vi "test_Multiple Global Type Cast Single Channel Command Message using Trigger and Padding.vi"(8 "error in (no error)":errorcluster, 11 "TestCase in":refnum<class "Instrument Addon Common System Tests.lvclass">) -> (0 "error out":errorcluster, 3 "TestCase out":refnum<class "Instrument Addon Common System Tests.lvclass">)   [LabVIEW 2019, in "Instrument Addon Common System Tests.lvclass"]
uses:
  Instrument Addon Common System Tests.lvclass
  C:/Program Files (x86)/National Instruments/LabVIEW 2019/vi.lib/NI/VeriStand Custom Device Testing Tools/VeriStandTestCase/VeriStandTestCase.lvclass
  <vilib>/NI VeriStand/Execution/Workspace/NI VeriStand - Set Multiple Channel Values.vi
  <vilib>/NI VeriStand/Execution/Workspace/NI VeriStand - Get Multiple Channel Values.vi
  <vilib>/addons/_JKI Toolkits/VI Tester/TestCase.llb/TestCase.lvclass
  <vilib>/NI VeriStand/Execution/Workspace/NI_VS Workspace ExecutionAPI.lvlib
  C:/Program Files (x86)/National Instruments/LabVIEW 2019/vi.lib/addons/_JKI Toolkits/VI Tester/TestCase.llb/TestCase.lvclass
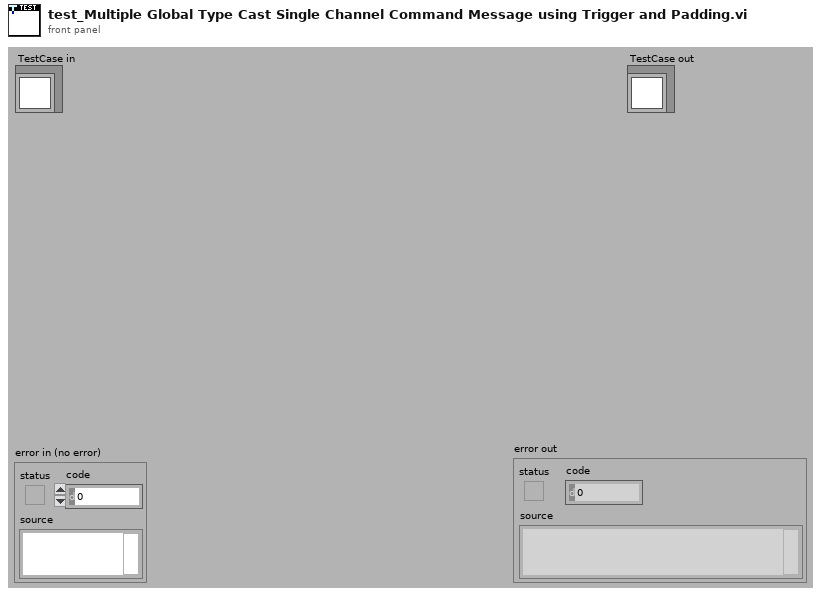
[diagram p1: front panel]
types:
  T1 = typedef "NI_VS Workspace ExecutionAPI.lvlib/WorkspaceAPI.ctl" = refnum<k24>
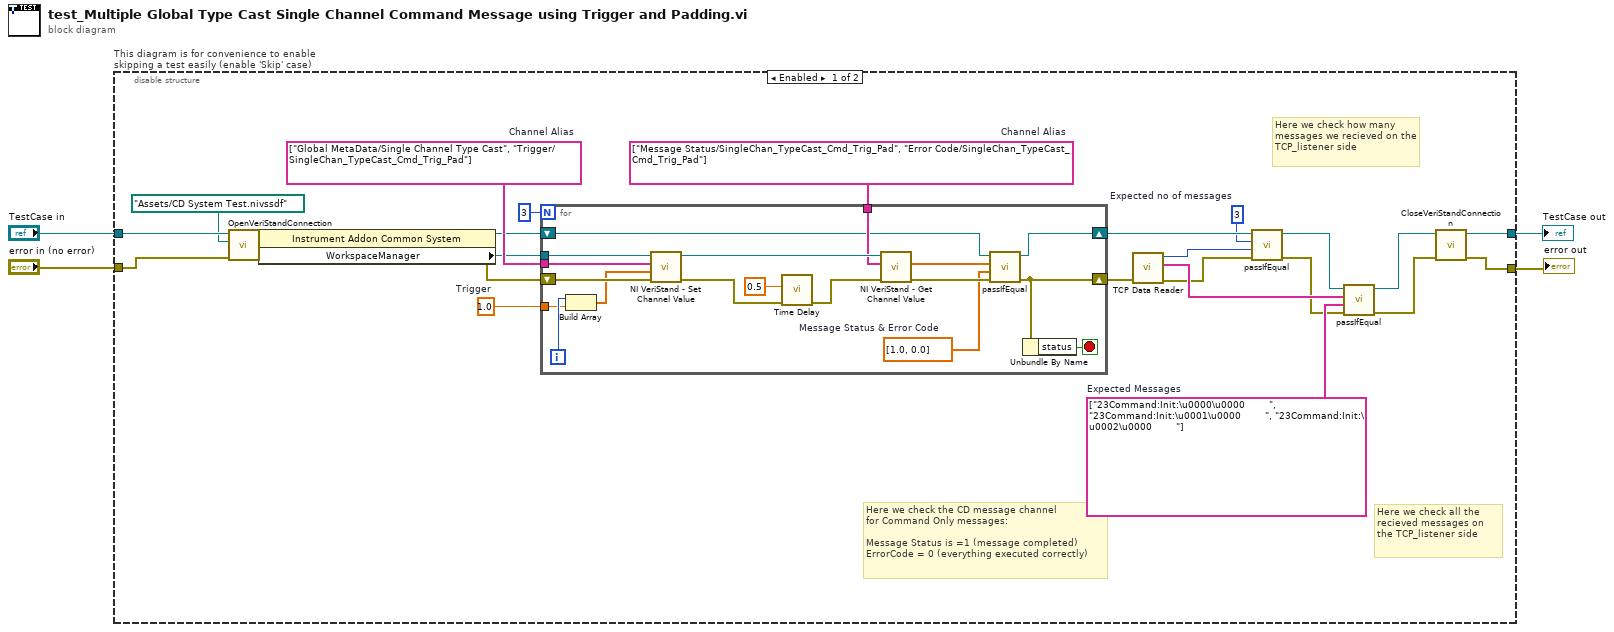
[diagram p0: block diagram]
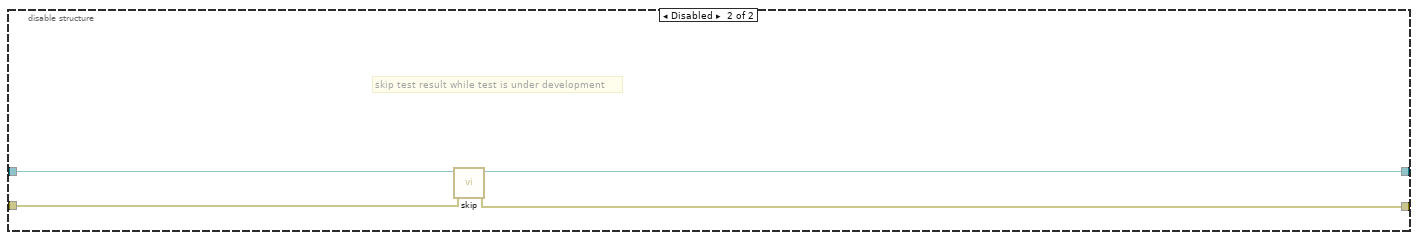
[diagram p2: hidden frame]
diagram:
  n1 = disable-structure "This diagram is for convenience to enable skipping a test easily (enable 'Skip' case)" shown="Enabled" {
    disable-tunnel: "TestCase in" -> [w27 w51]
    disable-tunnel: [w28 w49] -> w1
    disable-tunnel: [w29 w50] -> w3
    disable-tunnel: "error in (no error)" -> [w25 w48]
    frame Enabled {
      w11 = string[] ["23Command:Init:\u0000\u0000        ", "23Command:Init:\u0001\u0000        ", "23Command:Init:\u0002\u0000        "]  # Expected Messages
      w14 = string[] ["Message Status/SingleChan_TypeCast_Cmd_Trig_Pad", "Error Code/SingleChan_TypeCast_Cmd_Trig_Pad"]  # Channel Alias
      w8 = 3  # Expected no of messages
      w20 = 1.0  # Trigger
      w21 = string[] ["Global MetaData/Single Channel Type Cast", "Trigger/SingleChan_TypeCast_Cmd_Trig_Pad"]  # Channel Alias
      # "Here we check all the recieved messages on the TCP_listener side"
      # "Here we check how many messages we recieved on the TCP_listener side"
      # "Here we check the CD message channel\nfor Command Only messages:\n\nMessage Status is =1 (message completed)\nErrorCode = 0 (everything executed correctly)"
      n2 = call-dynamic "OpenVeriStandConnection.vi"("error in (no error)"=w25, "System Definition File"=path "Assets/CD System Test.nivssdf", "VeriStand Test Case in"=w27) -> ("error out"=w24:errorcluster, "VeriStand Test Case out"=w26:refnum<class "Instrument Addon Common System Tests.lvclass">)  [unwired: 6 in, 1 out]
      n3 = property class="Instrument Addon Common System "(reference=w26, error in=w24) -> (reference out=w18:refnum<class "Instrument Addon Common System Tests.lvclass">, error out=w22:errorcluster, "WorkspaceManager"=w7:T1)
      n4 = for {
        N: 3 -> [_]
        tunnel: w7 -> [w47]
        tunnel: w21 -> [w45]
        tunnel: w20 -> [w31]
        shift-right: [w34] -> w12
        shift-left: w22 -> [w46]
        tunnel: w14 -> [w43]
        shift-right: [w38] -> w13
        shift-left: w18 -> [w39]
        i -> [w32]
        stop <- w33 stop-if-true
        w35 = dbl[] [1.0, 0.0]  # Message Status & Error Code
        n5 = Build Array(w32, w31) -> (w30:dbl[])
        n6 = call-poly <vilib>:"NI VeriStand - Set Channel Value.vi"("error in (no error)"=w46, "Values"=w30, "Channels"=w45, "WorkspaceManager in"=w47) -> ("error out"=w41:errorcluster, "WorkspaceManager out"=w44:T1)  [unwired: 6 in]
        n7 = call "Time Delay"("error in (no error)"=w41, "Delay Time (s)"=0.5) -> ("error out"=w40:errorcluster)  [unwired: 9 in]
        n8 = call-poly <vilib>:"NI VeriStand - Get Channel Value.vi"("error in (no error)"=w40, "Channels"=w43, "WorkspaceManager in"=w44) -> ("error out"=w37:errorcluster, "Values"=w36:dbl[])  [unwired: 6 in, 1 out]
        n9 = call-dynamic "passIfEqual.vi"("error in (no error)"=w37, "y"=w35, "x"=w36, "TestCase in"=w39) -> ("error out"=w34:errorcluster, "TestCase out"=w38:refnum<class "Instrument Addon Common System Tests.lvclass">)  [unwired: 6 in]
        n10 = Unbundle By Name(w34) -> ("status"=w33:bool)
      }
      n11 = call "TCP Data Reader.vi"("error in (no error)"=w12) -> ("error out"=w5:errorcluster, "Recieved Messages"=w10:string[], "No of messages"=w9:i32)  [unwired: 8 in]
      n12 = call-dynamic "passIfEqual.vi"("error in (no error)"=w5, "y"=w9, "x"=w8, "TestCase in"=w13) -> ("error out"=w6:errorcluster, "TestCase out"=w17:refnum<class "Instrument Addon Common System Tests.lvclass">)  [unwired: 6 in]
      n13 = call-dynamic "passIfEqual.vi"("error in (no error)"=w6, "y"=w11, "x"=w10, "TestCase in"=w17) -> ("error out"=w15:errorcluster, "TestCase out"=w16:refnum<class "Instrument Addon Common System Tests.lvclass">)  [unwired: 6 in]
      n14 = call-dynamic "CloseVeriStandConnection.vi"("error in (no error)"=w15, "VeriStand Test Case in"=w16) -> ("error out"=w29:errorcluster, "VeriStand Test Case out"=w28:refnum<class "Instrument Addon Common System Tests.lvclass">)  [unwired: 8 in]
    }
    frame Disabled {
      # "skip test result while test is under development"
      n15 = call <vilib>:"skip.vi"("error in (no error)"=w48, "TestCase in"=w51) -> ("error out"=w50:errorcluster, "TestCase out"=w49:refnum<class "Instrument Addon Common System Tests.lvclass">)  [unwired: 8 in]
    }
  }
  "error out" <- w3
  "TestCase out" <- w1
